vi "ASK_PCM.vi"(9 "voice_path":string, 11 "PathIn":path) -> (0 "error out":errorcluster caption="错误输出", 1 "Origin_Bit":dbl[](array[numeric]) format="%#_13g", 3 "PathOut":path, 4 "Fs":dbl format="%#_13g")   [LabVIEW 2015]
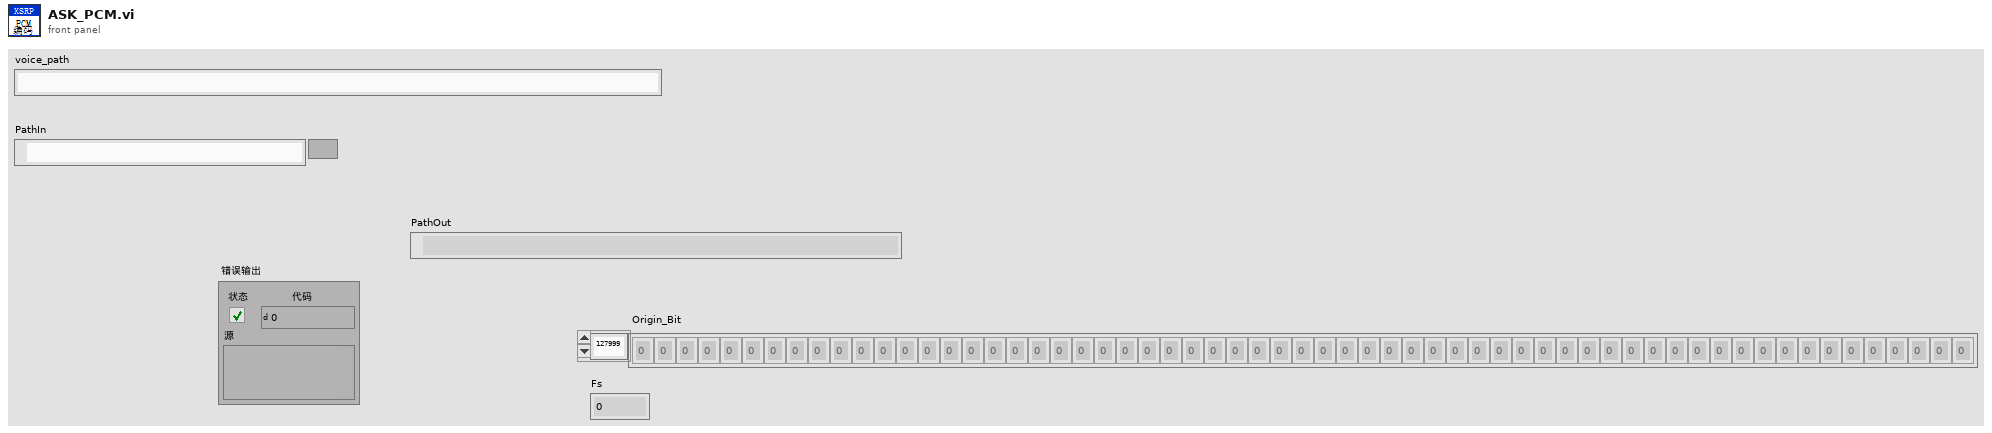
[diagram p1: front panel]
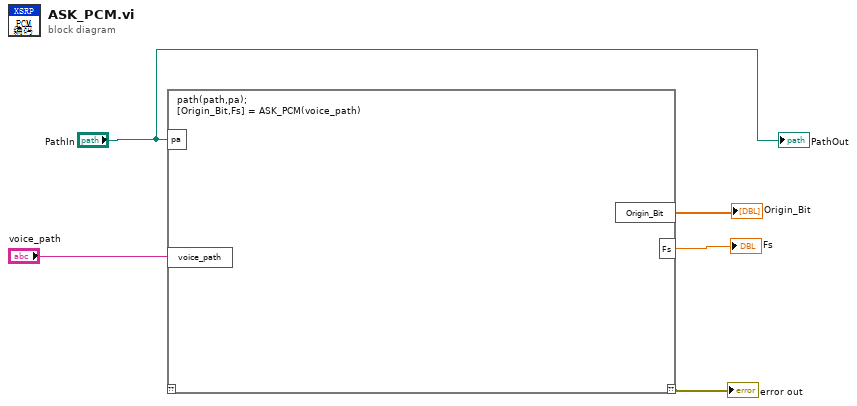
[diagram p0: block diagram]
diagram:
  n1 = script code="path(path,pa);\n[Origin_Bit,Fs] = ASK_PCM(voice_path)"("pa"="PathIn", "voice_path"="voice_path") -> ("??"=→"error out":errorcluster, "Origin_Bit"=→"Origin_Bit":dbl[], "Fs"=→"Fs":dbl)  [unwired: 1 in]
  "PathOut" <- "PathIn"
